vi "Serialize - JSON.vi"(8 "error in":errorcluster, 11 "humData in":refnum<class "humData.lvclass">) -> (0 "error out":errorcluster, 2 "Serialized JSON":string, 3 "humData out":refnum<class "humData.lvclass">)   [LabVIEW 2014, in "humData.lvclass"]
uses:
  humData.lvclass
  humData.lvclass/humData.ctl
  reusable/Data/Data.lvclass/Data.ctl
  reusable/Data/Read Data ID.vi
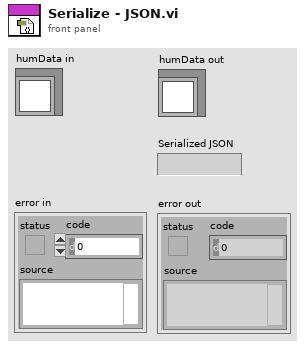
[diagram p1: front panel]
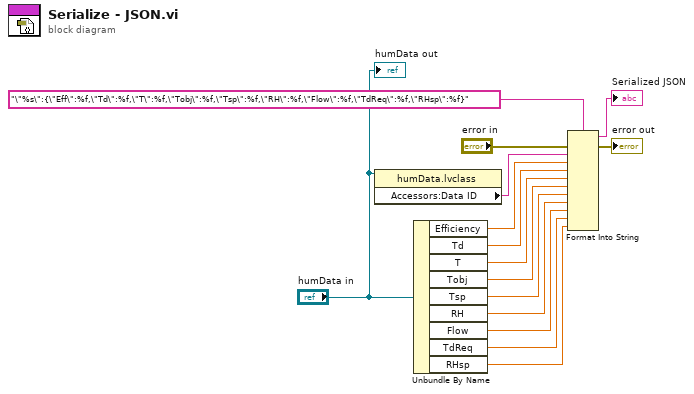
[diagram p0: block diagram]
diagram:
  n1 = property class="humData.lvclass"(reference="humData in") -> ("Accessors:Data ID"=w3:string)  [unwired: 1 in, 2 out]
  n2 = Unbundle By Name("humData in") -> ("Efficiency"=w4:dbl, "Td"=w14:dbl, "T"=w13:dbl, "Tobj"=w12:dbl, "Tsp"=w11:dbl, "RH"=w10:dbl, "Flow"=w9:dbl, "TdReq"=w2:dbl, "RHsp"=w1:dbl)
  n3 = Format Into String(format string="\"%s\":{\"Eff\":%f,\"Td\":%f,\"T\":%f,\"Tobj\":%f,\"Tsp\":%f,\"RH\":%f,\"Flow\":%f,\"TdReq\":%f,\"RHsp\":%f}", error in="error in", w3, w4, w14, w13, w12, w11, w10, w9, w2, w1) -> (resulting string=→"Serialized JSON":string, error out=→"error out":errorcluster)  [unwired: 1 in]
  "humData out" <- "humData in"
